vi "Calculate acceptance angle.vi"(8 "error in (no error)":errorcluster, 10 "Objective":string, 11 "FOV (true)":sgl) -> (0 "error out":errorcluster, 3 "Acceptance Angle (mrad)":dbl)   [LabVIEW 2017]
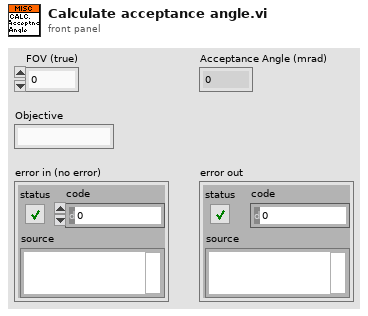
[diagram p1: front panel]
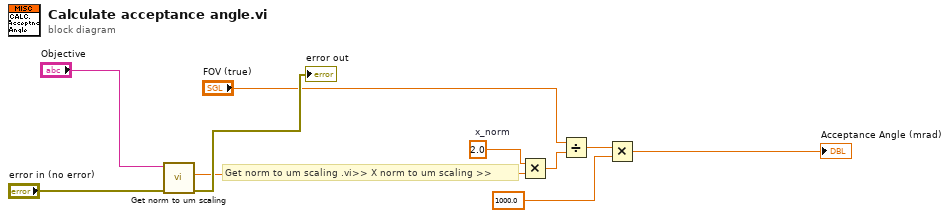
[diagram p0: block diagram]
diagram:
  w3 = 2.0  # x_norm
  # "Get norm to um scaling .vi>> X norm to um scaling >>"
  n1 = call "Get norm to um scaling .vi"("error in (no error)"="error in (no error)", "Current Objective"="Objective") -> ("error out"=→"error out":errorcluster, "X_norm to um_scaling"=w1:dbl)  [unwired: 7 in, 1 out]
  n2 = Multiply(x=w3, y=w1) -> (x*y=w2:dbl)
  n3 = Divide(x="FOV (true)", y=w2) -> (x/y=w4:dbl)
  n4 = Multiply(x=w4, y=1000.0) -> (x*y=→"Acceptance Angle (mrad)":dbl)
